vi "Vision Research Phantom Series PhCon PhSet.vi"(0 "CN [in]":u32, 1 "Sel":T1 items=["gsHasMechanicalShutter"=1025, "gsHasBlackLevel4"=1027, "gsHasCardFlash"=1051, "gsHas10G"=2000, "gsSupportsInternalBlackRef"=1026, "gsSupportsImageTrig"=1040, "gsSupportsCardFlash"=1050, "gsSupportsMagazine"=8193, "gsSupportsHQMode"=8194, "gsSupportsGenlock"=8195, "gsSupportsEDR"=8196, "gsSupportsAutoExposure"=8197, "gsSupportsTurbo"=8198, "gsSupportsBurstMode"=8199, "gsSupportsShutterOff"=8200, "gsSupportsDualSDIOutput"=8201, "gsSupportsRecordingCines"=8202, "gsSupportsV444"=8203, "gsSupportsInterlacedSensor"=8204, "gsSupportsRampFRP"=8205, "gsSensorTemperature"=1028, "gsCameraTemperature"=1029, "gsThermoElectricPower"=1030, "gsSensorTemperatureThreshold"=1031, "gsCameraTemperatureThreshold"=1032, "gsVideoPlayCine"=1033, "gsVideoPlaySpeed"=1034, "gsVideoOutputConfig"=1035, "gsMechanicalShutter"=1036, "gsImageTrigThreshold"=1041, "gsImageTrigAreaPercentage"=1042, "gsImageTrigSpeed"=1043, "gsImageTrigMode"=1044, "gsImageTrigRect"=1045, "gsAutoProgress"=1046, "gsAutoBlackRef"=1047, "gsCardFlashSizeK"=1052, "gsCardFlashFreeK"=1053, "gsCardFlashError"=1054, "gsEthernetAddress"=1055, "gsEthernetMask"=1056, "gsEthernetBroadcast"=1057, "gsEthernetGateway"=1058, "gsLensFocus"=1059, "gsLensAperature"=1060, "gsLensAperatureRange"=1061, "gsLensDescription"=1062, "gsLensFocusInProgress"=1063, "gsLensFocusAtLimit"=1064, "gsGenlock"=1065, "gsGenlockStatus"=1066, "gsTurboMode"=1068, "gsModel"=1069, "gsIPAddress"=1070], 2 "pVal [in]":u64, 5 "Error In (no error)":errorcluster) -> (14 "CN [out]":u32=1, 15 "pVal [out]":u64, 19 "Error Out":errorcluster)   [LabVIEW 2013, in "VRI.lvlib"]
doc: "PhSet\nHRESULT PhSet(UNIT CN, UINT Sel, PVOID pVal)\n\nParameters\nCN [in]\n Camera number.\nSel [in]\n Selection value indicating information to be set.\npVal [out]\n Pointer to the buffer containing data to be set.\n \nReturn Value\nThe function returns ERR_Ok in case of success or an error code, otherwise. To get extended error information call PhGetErrorMessage.\n\nRemarks\nThis function performs a set operation for the given camera.\nFor a complete list of currently available selectors, go to Appendix 2.\nPlease note that the last parameter must be passed by reference. The function will return back to the called the value actually accepted for the specified parameter.\n\nRequired Header\nPhCon.h"
uses:
  VRI.lvlib
  _Type Defs/PhCon GS.ctl
  Phantom DLLs/PhCon.dll
panel:
  # "For instructions on the use of this VI, press Ctrl+H to display the help window and move the mouse over the icon, controls, and indicators"
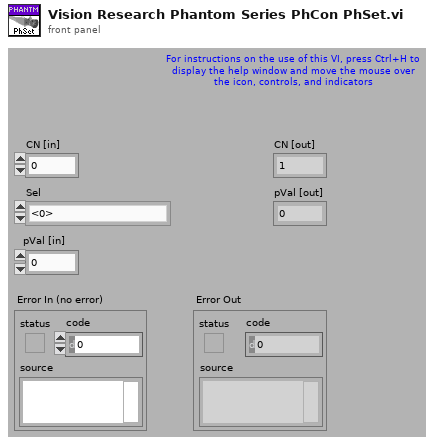
[diagram p1: front panel]
types:
  T1 = typedef "VRI.lvlib/PhCon GS.ctl" = u16
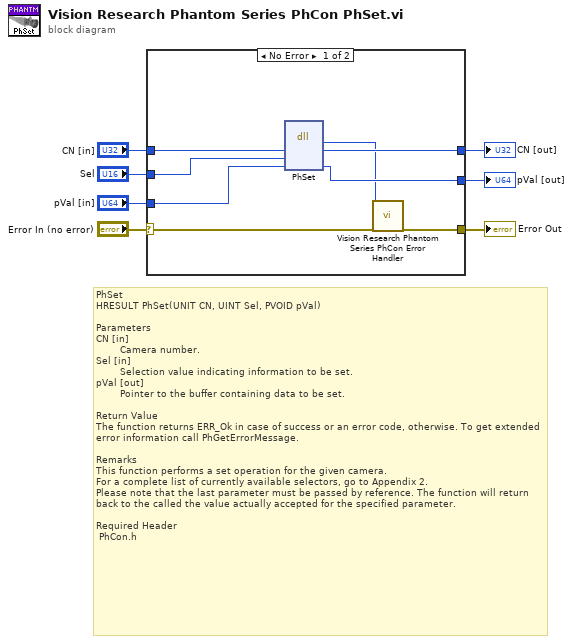
[diagram p0: block diagram]
diagram:
  # "PhSet\nHRESULT PhSet(UNIT CN, UINT Sel, PVOID pVal)\n\nParameters\nCN [in]\n\t       Camera number.\nSel [in]\n\t       Selection value indicating information to be set.\npVal [out]\n\t       Pointer to the buffer containing data to be set.\n \nReturn Value\nThe function returns ERR_Ok in case of success or an error code, otherwise. To get extended error information call PhGetErrorMessage.\n\nRemarks\nThis function performs a set operation for the given camera.\nFor a complete list of currently available selectors, go to Appendix 2.\nPlease note that the last parameter must be passed by reference. The function will return back to the called the value actually accepted for the specified parameter.\n\nRequired Header\n\tPhCon.h"
  n1 = case shown="No Error" "Error In (no error)" {
    selector: "Error In (no error)" -> [w15 w18]
    tunnel: [w14 w18] -> w6
    tunnel: "CN [in]" -> [w13 w17]
    tunnel: [w12 w17] -> w4
    tunnel: "Sel" -> [w11 _]
    tunnel: "pVal [in]" -> [w10 w16]
    tunnel: [w9 w16] -> w1
    frame No Error {
      n2 = dll-call lib="C:/Projects/SDK/32-bit/Vision Research Phantom Series Labview Driver/Phantom DLLs/PhCon.dll" fn="PhSet"("CN"=w13, "Sel"=w11, "pVal"=w10) -> ("HRESULT"=w8:i32, "CN"=w12:u32, "pVal"=w9:u64)  [unwired: 3 in, 3 out]
      n3 = call "Vision Research Phantom Series PhCon Error Handler.vi"("ErrNo"=w8, "Error In (no error)"=w15) -> ("Error Out"=w14:errorcluster)  [unwired: 17 out]
    }
    frame Error {
    }
  }
  "Error Out" <- w6
  "CN [out]" <- w4
  "pVal [out]" <- w1
